vi "Get-correlation-image-shift.vi"(8 "error in":errorcluster, 11 "Data ref. in":refnum<data-value>) -> (0 "error IO":errorcluster, 1 "Y-shift":i32, 2 "X-shift":i32, 3 "Data ref.":refnum<data-value>)   [LabVIEW 2013, in "CameraVision.lvlib" / "CV-Main.lvclass"]
uses:
  CV-Main.lvclass
  CV-Main.lvclass/CV-Main.ctl
  Correction/CV-Correction.lvclass/CV-Correction.ctl
  Read Correct params.vi
  Correction/Read X-shift.vi
  Correction/Read Y-shift.vi
  Correction/CV-Correction.lvclass
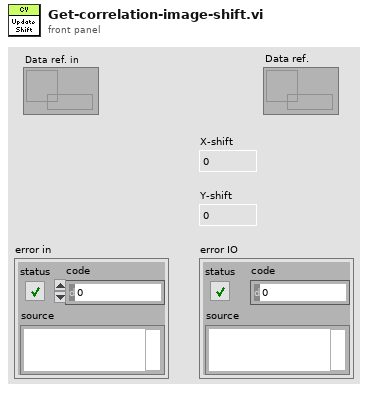
[diagram p1: front panel]
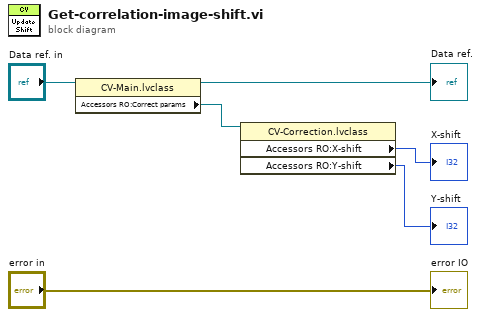
[diagram p0: block diagram]
diagram:
  n1 = property class="CV-Main.lvclass"(reference="Data ref. in") -> (reference out=→"Data ref.":refnum<data-value>, "Accessors RO:Correct params"=w1:refnum<data-value>)  [unwired: 1 in, 1 out]
  n2 = property class="CV-Correction.lvclass"(reference=w1) -> ("Accessors RO:X-shift"=→"X-shift":i32, "Accessors RO:Y-shift"=→"Y-shift":i32)  [unwired: 1 in, 2 out]
  "error IO" <- "error in"
